vi "tagDB_IsValid.vi"(8 "error in (no error)":errorcluster, 11 "DB Ref in":T1) -> (0 "error out":errorcluster, 2 "valid?":bool, 3 "DB Ref out":T1)   [LabVIEW 2014, in "TagDB(dev).lvlib"]
doc: "[Covers: REQ_API_ISVALID]"
uses:
  TagDB(dev).lvlib
  tagDB_Def.ctl
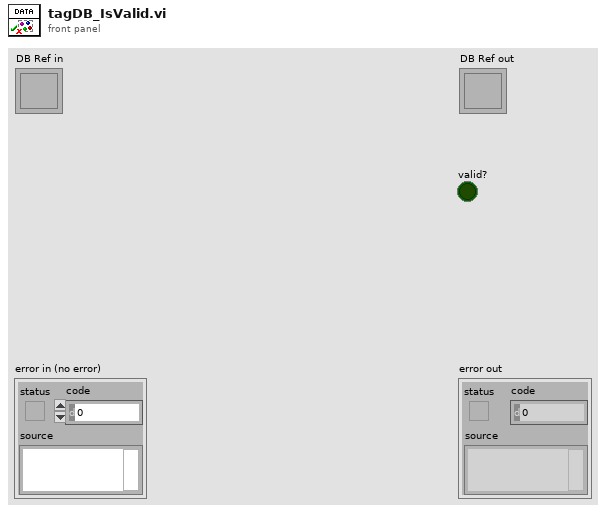
[diagram p1: front panel]
types:
  T1 = typedef "TagDB(dev).lvlib/tagDB_Def.ctl" = refnum<k1>
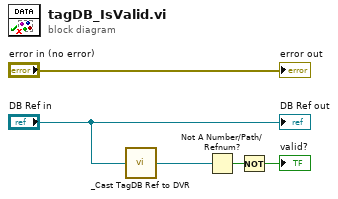
[diagram p0: block diagram]
diagram:
  n1 = call "_Cast TagDB Ref to DVR.vi"("TagDB"="DB Ref in") -> ("DVR"=w2:refnum<data-value>)  [unwired: 4 in]
  n2 = Not A Number/Path/Refnum?(number/path/refnum=w2) -> (NaN/Path/Refnum?=w1:bool)
  n3 = Not(x=w1) -> (.not. x?=→"valid?":bool)
  "error out" <- "error in (no error)"
  "DB Ref out" <- "DB Ref in"
